vi "Find Sink To Source Terminal.vi"(0 "Source Terminal":refnum<vi>, 11 "error in (no error)":errorcluster) -> (4 "Sink Terminal":refnum<vi>, 15 "error out":errorcluster)   [LabVIEW 2019, in "MVA Message Mapper.lvlib"]
uses:
  MVA Message Mapper.lvlib
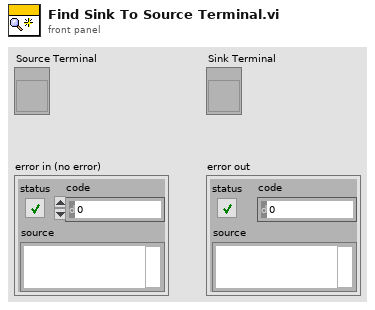
[diagram p1: front panel]
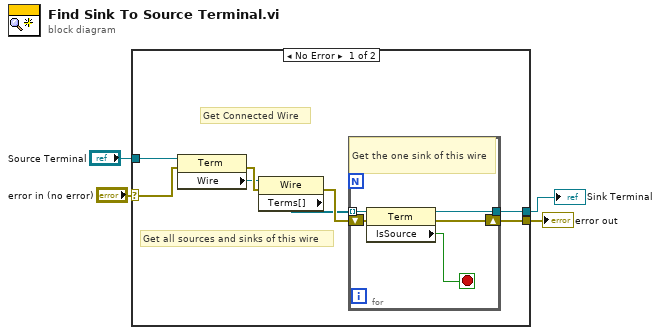
[diagram p0: block diagram]
diagram:
  n1 = case shown="No Error" "error in (no error)" {
    selector: "error in (no error)" -> [w8 w18]
    tunnel: [w12 w18] -> w4
    tunnel: [w11 _] -> w1
    tunnel: "Source Terminal" -> [w5 _]
    frame No Error {
      # "Get Connected Wire"
      # "Get all sources and sinks of this wire"
      n2 = property on="Property Node" class="Term"(reference=w5, error in=w8) -> (error out=w9:errorcluster, "Wire"=w7:refnum<vi>)  [unwired: 1 out]
      n3 = property on="Property Node" class="Wire"(reference=w7, error in=w9) -> (error out=w10:errorcluster, "Terms[]"=w6:refnum<vi>[])  [unwired: 1 out]
      n4 = for {
        tunnel: w6 -> [w17] mode=indexing
        tunnel: [w15] -> w11
        shift-right: [w13] -> w12
        shift-left: w10 -> [w14]
        stop <- w16 stop-if-true
        # "Get the one sink of this wire"
        n5 = property class="Term"(reference=w17, error in=w14) -> (reference out=w15:refnum<vi>, error out=w13:errorcluster, "IsSource"=w16:bool)
      }
    }
    frame Error {
    }
  }
  "error out" <- w4
  "Sink Terminal" <- w1
